vi "CliGetOrderCode.vi"(0 "ref in":u64, 11 "error in (no error)":errorcluster) -> (2 "OrderCode":string, 4 "ref out":u64, 6 "Result":i32, 12 "V3":u8, 13 "V2":u8, 14 "V1":u8, 15 "error out":errorcluster)   [LabVIEW 2018, in "Snap7.lvlib"]
uses:
  Snap7.lvlib
  windows/lv_snap7.dll
panel:
  in  "V3_var":u8
  in  "V2_var":u8
  in  "V1_var":u8
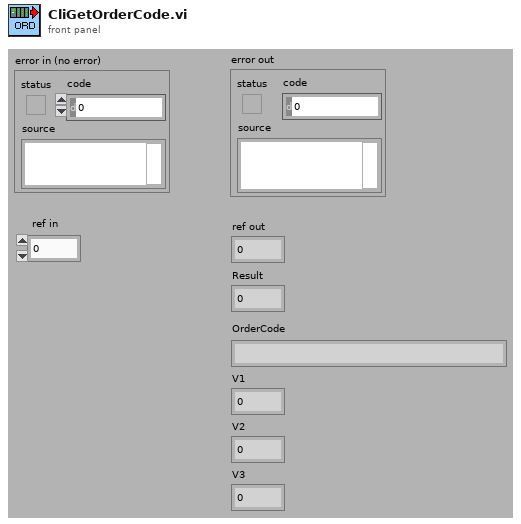
[diagram p1: front panel]
types:
  T1 = enum16{"big-endian, network order", "native, host order", "little-endian"}
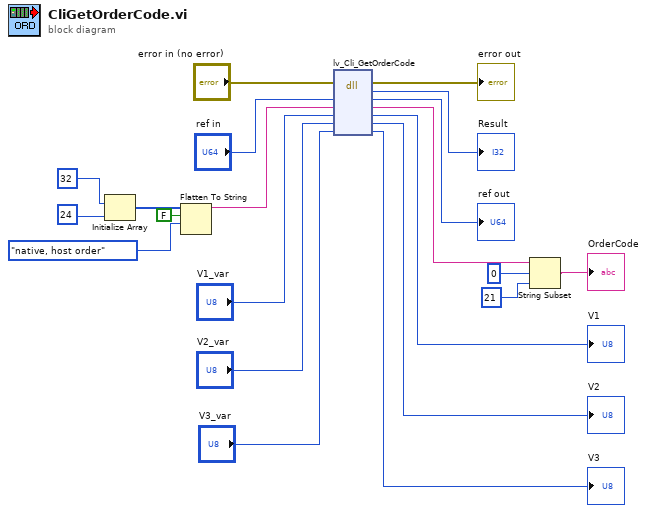
[diagram p0: block diagram]
diagram:
  n1 = Initialize Array(u8 32, 24) -> (w17:u8[])
  n2 = Flatten To String(anything=w17, prepend array or string size? (T)=FALSE, byte order (0:big-endian, network order)=T1."native, host order") -> (data string=w9:string)  [unwired: 1 in, 2 out]
  n3 = dll-call lib="C:/Users/WanLiMing/Downloads/snap7-full-1.4.2/snap7-full-1.4.2/LabVIEW/lib/windows/lv_snap7.dll" fn="lv_Cli_GetOrderCode"(error in="error in (no error)", "Client"="ref in", "StringData"=w9, "V1"="V1_var", "V2"="V2_var", "V3"="V3_var") -> (error out=→"error out":errorcluster, "return type"=→"Result":i32, "Client"=→"ref out":u64, "StringData"=w4:string, "V1"=→"V1":u8, "V2"=→"V2":u8, "V3"=→"V3":u8)  [unwired: 2 in, 1 out]
  n4 = String Subset(string=w4, offset (0)=0, length (rest)=21 ("length (rest)")) -> (substring=→"OrderCode":string)
